vi "FA_ConvertToAgentConfig.vi"(8 "Error In":errorcluster, 11 "Config":T1) -> (0 "Error Out":errorcluster, 3 "AgentConfig":T3)   [LabVIEW 2014, in "FA_AgentConfig.lvlib"]
doc: "Coverts FA_NativeType's Config control to AgentConfig Special Type control."
uses:
  FA_AgentConfig.lvlib
  FA_AgentConfig.ctl
  FA_NativeTypes API/source/VI Source/FA_Config.ctl
  FA_LocalStore API/source/VI Source/FA_LSSpecialTypes.ctl
  FA_LocalStore API/source/VI Source/FA_LocalStore.lvlib
  FA_NativeTypes API/source/VI Source/FA_NativeTypes.lvlib
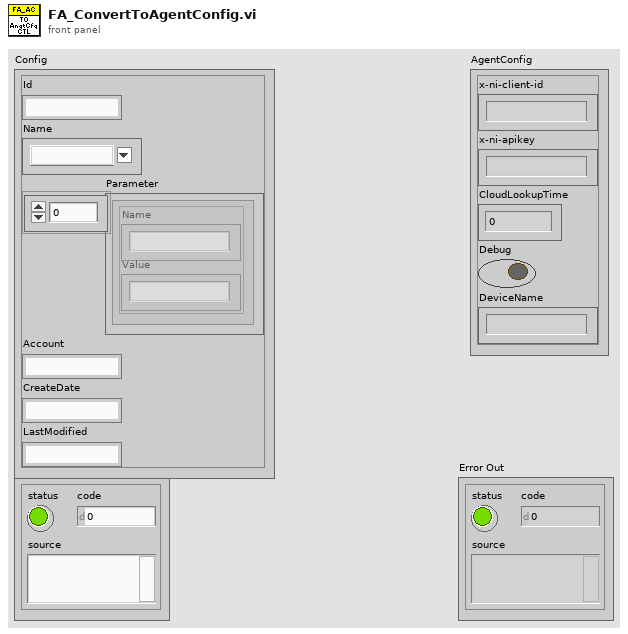
[diagram p1: front panel]
types:
  T1 = typedef "FA_NativeTypes.lvlib/FA_Config.ctl" = cluster{"Id":string, "Name":T2, "Parameter":cluster{"Name":string, "Value":string}[], "Account":string, "CreateDate":string, "LastModified":string}
  T2 = typedef "FA_LocalStore.lvlib/FA_LSSpecialTypes.ctl" = string
  T3 = typedef "FA_AgentConfig.lvlib/FA_AgentConfig.ctl" = cluster{"x-ni-client-id":string, "x-ni-apikey":string, "CloudLookupTime":u32, "Debug":bool, "DeviceName":string}
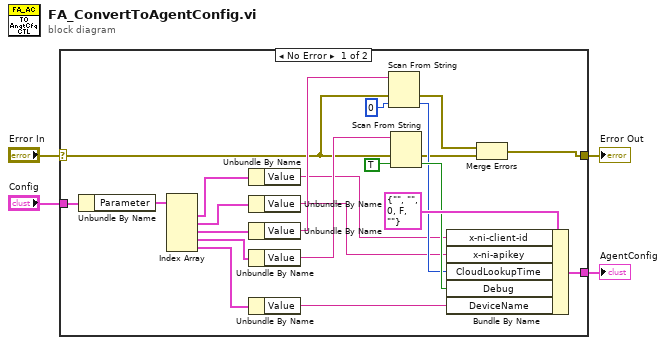
[diagram p0: block diagram]
diagram:
  n1 = case shown="No Error" "Error In" {
    selector: "Error In" -> [w13 w27]
    tunnel: [w10 w27] -> w4
    tunnel: "Config" -> [w26 _]
    tunnel: [w7 _] -> w1
    frame No Error {
      n2 = Unbundle By Name(w26) -> ("Parameter"=w25:cluster{"Name":string, "Value":string}[])
      n3 = Index Array(array=w25) -> (element #1=w24:cluster{"Name":string, "Value":string}, element #2=w23:cluster{"Name":string, "Value":string}, element #3=w22:cluster{"Name":string, "Value":string}, element #4=w21:cluster{"Name":string, "Value":string}, element #5=w6:cluster{"Name":string, "Value":string})  [unwired: 5 in]
      n4 = Unbundle By Name(w24) -> ("Value"=w9:string)
      n5 = Unbundle By Name(w23) -> ("Value"=w8:string)
      n6 = Unbundle By Name(w22) -> ("Value"=w20:string)
      n7 = Unbundle By Name(w21) -> ("Value"=w17:string)
      n8 = Unbundle By Name(w6) -> ("Value"=w5:string)
      n9 = Scan From String(input string=w20, error in=w13, default 1=u32 0) -> (error out=w12:errorcluster, output 1=w14:u32)  [unwired: 2 in, 2 out]
      n10 = Scan From String(input string=w17, error in=w13, default 1=TRUE) -> (error out=w11:errorcluster, output 1=w15:bool)  [unwired: 2 in, 2 out]
      n11 = Bundle By Name(cluster=T3 {"x-ni-client-id"="", "x-ni-apikey"="", "CloudLookupTime"=0, "Debug"=FALSE, "DeviceName"=""} ("AgentConfig"), "x-ni-client-id"=w9, "x-ni-apikey"=w8, "CloudLookupTime"=w14, "Debug"=w15, "DeviceName"=w5) -> (w7:T3)
      n12 = Merge Errors(w12, w11) -> (w10:errorcluster)
    }
    frame Error {
    }
  }
  "Error Out" <- w4
  "AgentConfig" <- w1
